vi "globalTearDown.vi"(8 "error in (no error)":errorcluster, 11 "MyFirstTest in":refnum<class "MyFirstTest.lvclass">) -> (0 "error out":errorcluster, 3 "MyFirstTest out":refnum<class "MyFirstTest.lvclass">)   [LabVIEW 2013, in "MyFirstTest.lvclass"]
uses:
  MyFirstTest.lvclass
panel:
  out "created new?":bool
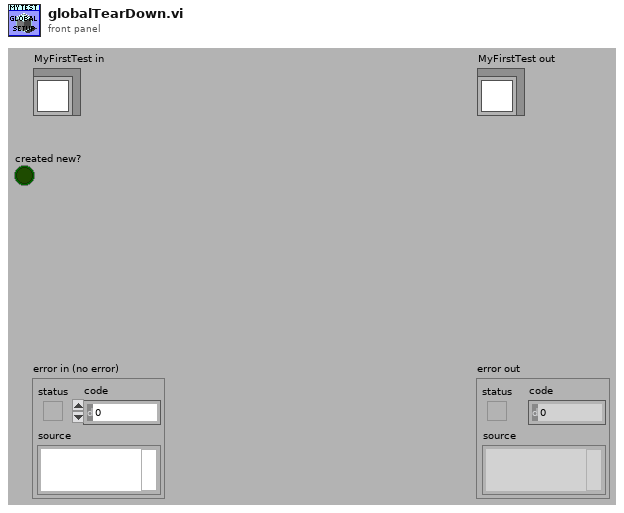
[diagram p1: front panel]
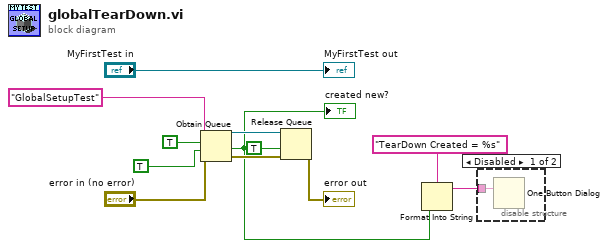
[diagram p0: block diagram]
diagram:
  n1 = Obtain Queue(name (unnamed)="GlobalSetupTest", element data type=TRUE, create if not found? (T)=TRUE, error in (no error)="error in (no error)") -> (queue out=w7:refnum<queue>, created new?=w2:bool, error out=w6:errorcluster)  [unwired: 1 in]
  "created new?" <- w2
  n2 = Release Queue(queue=w7, force destroy? (F)=TRUE, error in (no error)=w6) -> (error out=→"error out":errorcluster)  [unwired: 2 out]
  n3 = Format Into String(format string="TearDown Created = %s", w2) -> (resulting string=w4:string)  [unwired: 2 in, 1 out]
  n4 = disable-structure shown="Disabled" {
    disable-tunnel: w4 -> [w13 _]
    frame Disabled {
      n5 = One Button Dialog(message=w13) -> ()  [unwired: 1 in, 1 out]
    }
    frame Enabled {
    }
  }
  "MyFirstTest out" <- "MyFirstTest in"
